vi "Test_MergeErrorsPublication_WarningCluster_WarningIgnored.vi"(8 "error in (no error)":errorcluster, 11 "TestCase in":refnum<class "TestPublicationPolicy.lvclass">) -> (0 "error out":errorcluster, 3 "TestCase out":refnum<class "TestPublicationPolicy.lvclass">)   [LabVIEW 2020, in "TestPublicationPolicy.lvclass"]
uses:
  TestPublicationPolicy.lvclass
  TestPublicationPolicy.lvclass/TestPublicationPolicy.ctl
  Source/IMediator/MutexedPublishRequest/MutexedPublishRequest.lvclass
  Source/IMediator/IPublicationPolicy/IPublicationPolicy.lvclass
  Source/PublicationPolicy/MergeErrorsPublication/MergeErrorsPublication.lvclass
  modules/composed-transport/Source/Concrete/NotifierTransport/NotifierTransport.lvclass
  C:/Git/mva-core/Source/IMediator/IPublicationPolicy/IPublicationPolicy.lvclass
  C:/Git/mva-core/Source/PublicationPolicy/MergeErrorsPublication/MergeErrorsPublication.lvclass
  C:/Git/mva-core/modules/composed-transport/Source/ITransport/ITransport.lvclass
  C:/Git/mva-core/modules/composed-transport/Source/Concrete/NotifierTransport/NotifierTransport.lvclass
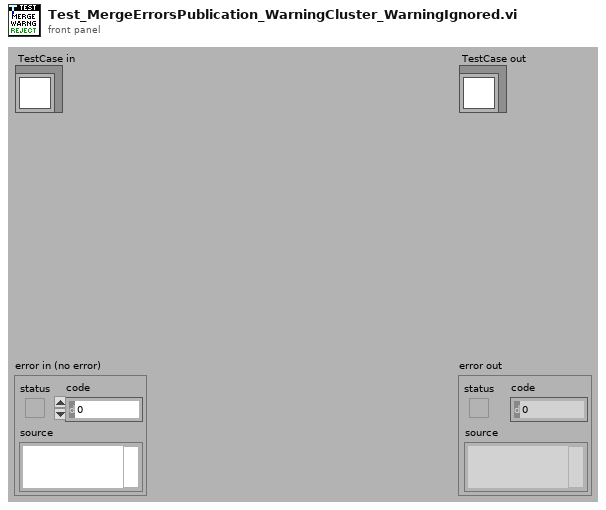
[diagram p1: front panel]
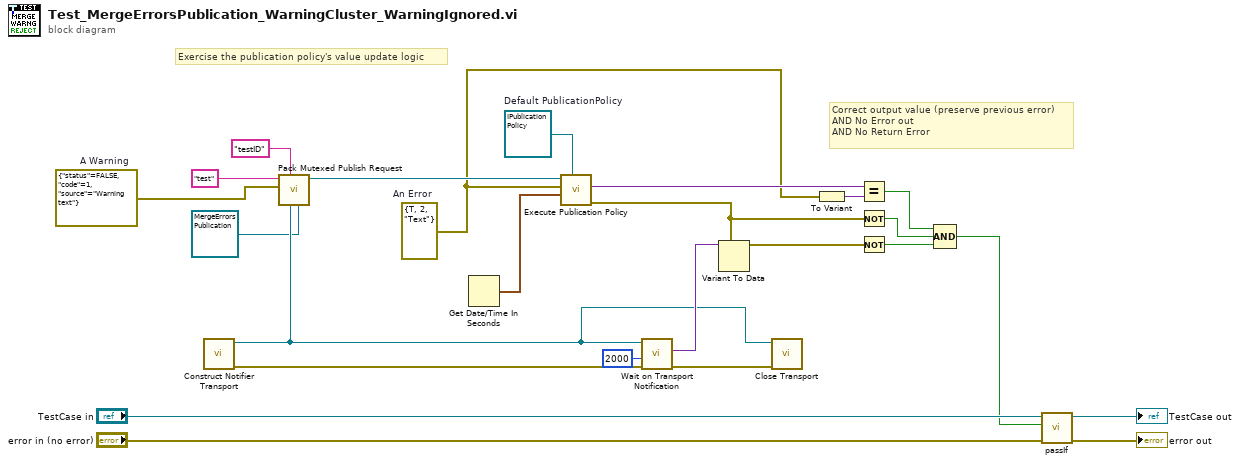
[diagram p0: block diagram]
diagram:
  w6 = errorcluster {"status"=FALSE, "code"=1, "source"="Warning text"}  # A Warning
  w19 = refnum<class "IPublicationPolicy.lvclass"> refnum  # Default PublicationPolicy
  w4 = errorcluster {"status"=TRUE, "code"=2, "source"="Text"}  # An Error
  # "Correct output value (preserve previous error)\nAND No Error out\nAND No Return Error"
  # "Exercise the publication policy's value update logic"
  n1 = call "Construct Notifier Transport.vi"() -> ("error out"=w16:errorcluster, "NotifierTransport"=w3:refnum<class "NotifierTransport.lvclass">)  [unwired: 10 in]
  n2 = call "Pack Mutexed Publish Request.vi"("PublicationPolicy"=refnum<class "MergeErrorsPublication.lvclass"> refnum ("PublicationPolicy.lvlib:MergeErrorsPublication.lvclass"), "Return Error Transport"=w3, "Publisher ID"="testID", "Datum Value or Type"=w6, "Datum Name"="test") -> ("MutexedPublishRequest Out"=w20:refnum<class "MutexedPublishRequest.lvclass">)  [unwired: 5 in, 1 out]
  n3 = Get Date/Time In Seconds() -> (seconds since 1Jan1904=w21:timestamp)
  n4 = call-dynamic "Execute Publication Policy.vi"("Default PublicationPolicy"=w19, "Last Publish Time"=w21, "Last Published Value"=w4, "MutexedPublishRequest"=w20) -> ("error out (Reject Publication)"=w8:errorcluster, "Value to Publish"=w13:variant)  [unwired: 5 in, 1 out]
  n5 = call "Wait on Transport Notification.vi"("error in (no error)"=w16, "Timeout In ms (-1)"=2000, "NotifierTransport"=w3) -> ("error out"=w2:errorcluster, "Data"=w14:variant)  [unwired: 6 in, 1 out]
  n6 = Variant To Data(type=w8, Variant=w14) -> (data=w11:errorcluster)  [unwired: 1 in, 1 out]
  n7 = call-dynamic "Close Transport.vi"("error in (no error)"=w2, "NotifierTransport"=w3) -> ()  [unwired: 9 in, 1 out]
  n8 = To Variant(anything=w4) -> (Variant=w12:variant)
  n9 = Equal?(x=w13, y=w12) -> (x = y?=w10:bool)
  n10 = Not(x=w8) -> (.not. x?=w7:bool)
  n11 = Not(x=w11) -> (.not. x?=w9:bool)
  n12 = Compound Arithmetic op=AND(w10, w7, w9) -> (w5:bool)
  n13 = call-dynamic "passIf.vi"("error in (no error)"="error in (no error)", "pass"=w5, "TestCase in"="TestCase in") -> ("error out"=→"error out":errorcluster, "TestCase out"=→"TestCase out":refnum<class "TestPublicationPolicy.lvclass">)  [unwired: 7 in]
